vi "Paint Bounding Box (3).vi"(9 "Camera Image":T3, 10 "R/G/B":cluster{"Lower value":i32, "Upper value":i32}[](array[cluster])=[{"Lower value"=0, "Upper value"=40}, {"Lower value"=80, "Upper value"=255}, {"Lower value"=0, "Upper value"=255}]) -> (0 "Thresholded Image":T3(plugin-control), 1 "Bounding Box Final":T4, 2 "Particle Report 2":T1, 3 "Particle Report":T1, 4 "General Report":T2(array[cluster]))   [LabVIEW 2016]
uses:
  <vilib>/vision/Image Controls.llb/IMAQ Image.ctl
panel:
  out "Particle Report":T2(array[cluster]) {"Orientation" format="%.2f"; "Dimensions"."Height" format="%.2f"; "Dimensions"."Width" format="%.2f"; "Center of Mass"."Y" format="%.2f"; "Center of Mass"."X" format="%.2f"; "Bounding Rect"."Bottom" format="%.2f"; "Bounding Rect"."Right" format="%.2f"; "Bounding Rect"."Top" format="%.2f"; "Bounding Rect"."Left" format="%.2f"; "Number of Holes" format="%.2f"; "Area" format="%.2f"}
  in  "sampleimage":string
  out "Base Image":T3(plugin-control)
  # "difference = width*4"
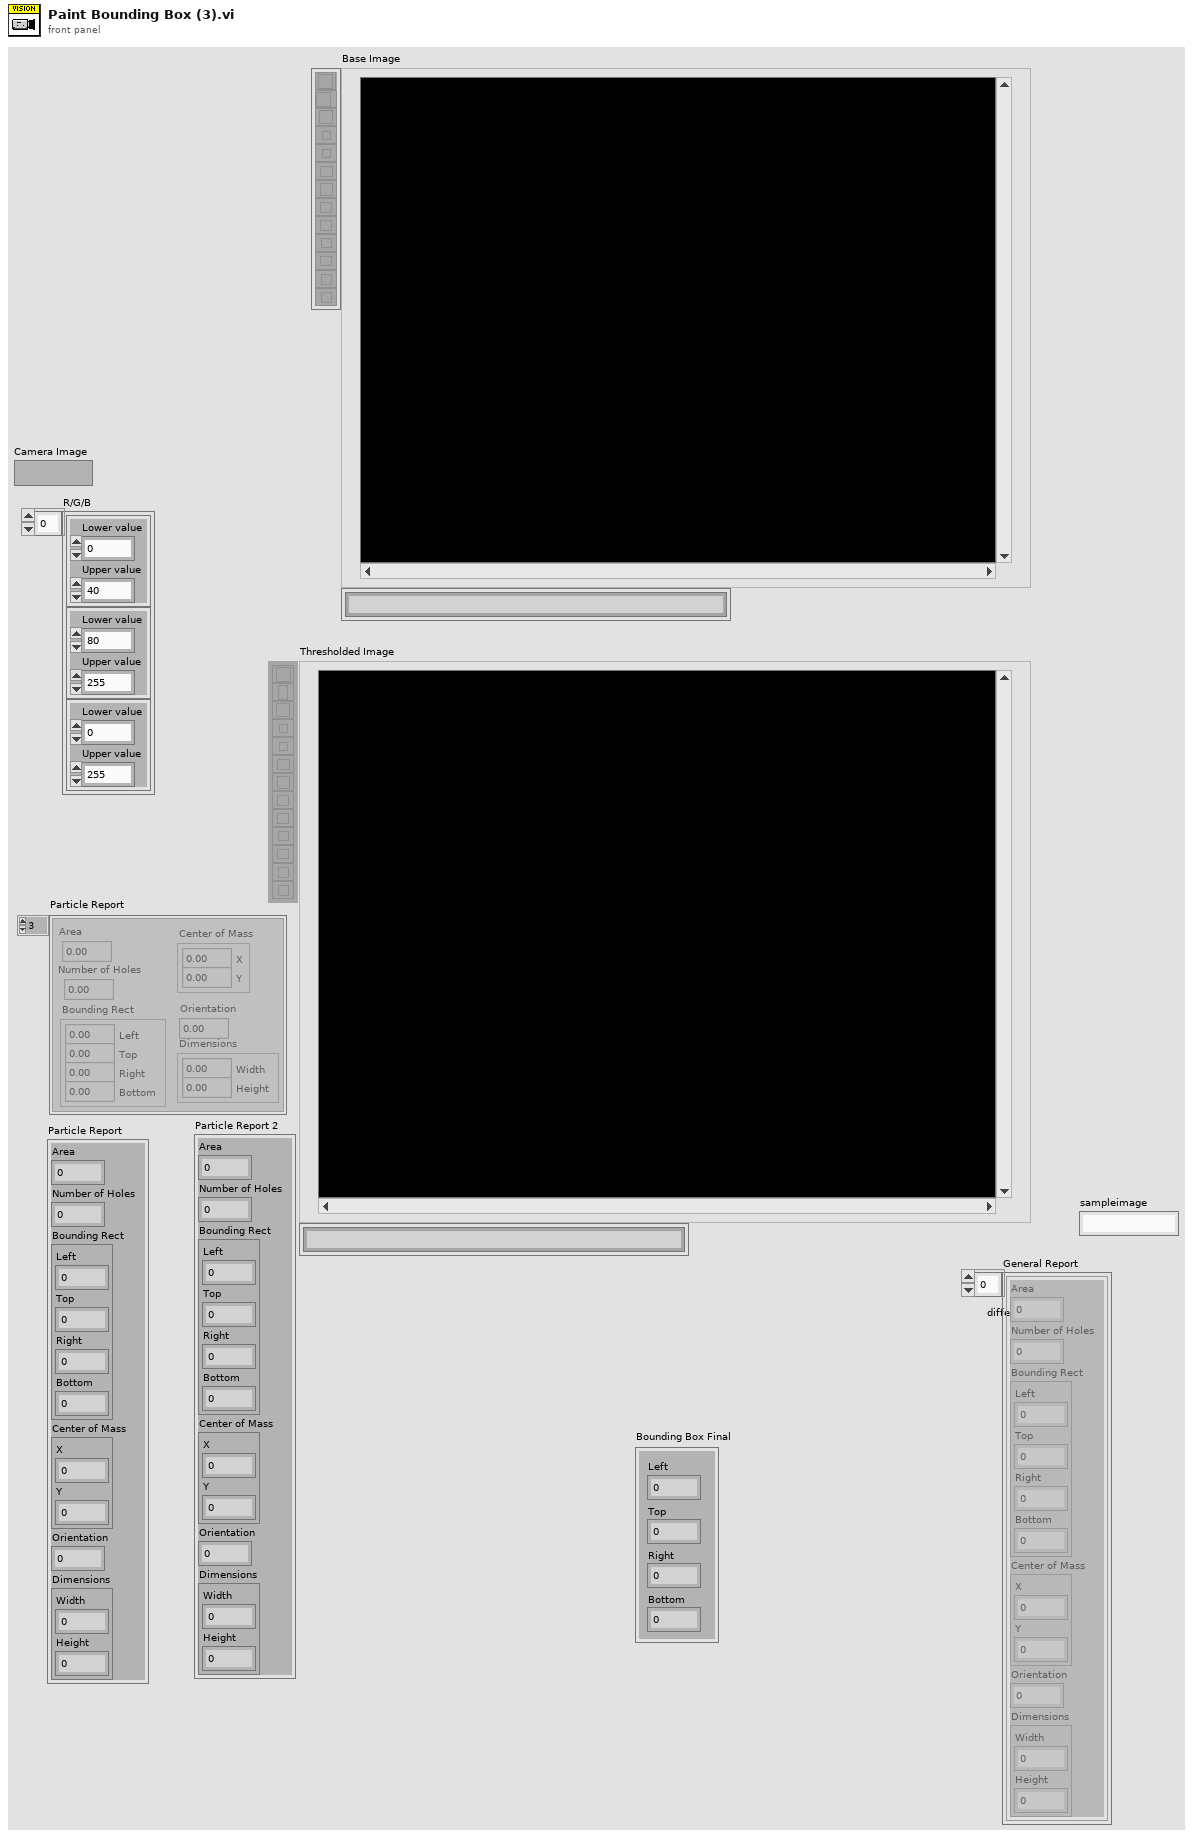
[diagram p1: front panel]
types:
  T1 = cluster{"Area":dbl, "Number of Holes":dbl, "Bounding Rect":cluster{"Left":dbl, "Top":dbl, "Right":dbl, "Bottom":dbl}, "Center of Mass":cluster{"X":dbl, "Y":dbl}, "Orientation":dbl, "Dimensions":cluster{"Width":dbl, "Height":dbl}}
  T2 = cluster{"Area":dbl, "Number of Holes":dbl, "Bounding Rect":cluster{"Left":dbl, "Top":dbl, "Right":dbl, "Bottom":dbl}, "Center of Mass":cluster{"X":dbl, "Y":dbl}, "Orientation":dbl, "Dimensions":cluster{"Width":dbl, "Height":dbl}}[]
  T3 = typedef "IMAQ Image.ctl" = refnum<image>
  T4 = cluster{"Left":dbl, "Top":dbl, "Right":dbl, "Bottom":dbl}
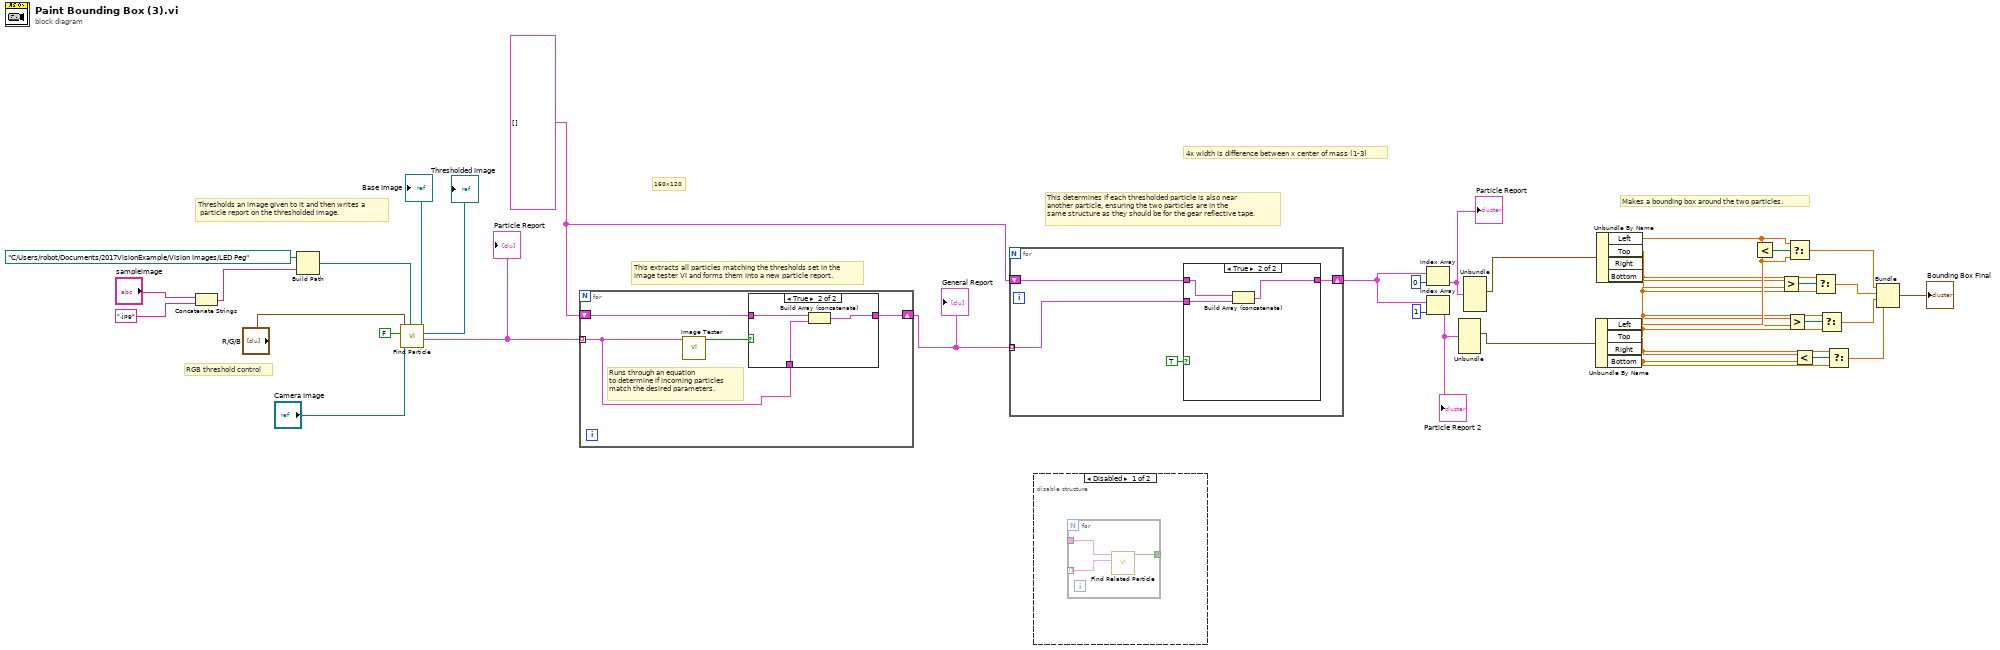
[diagram p0: block diagram]
diagram:
  w3 = T2 []
  # "This determines if each thresholded particle is also near \nanother particle, ensuring the two particles are in the \nsame structure as they should be for the gear reflective tape."
  # "Makes a bounding box around the two particles."
  # "4x width is difference between x center of mass (1-3)"
  # "RGB threshold control"
  # "This extracts all particles matching the thresholds set in the \nimage tester VI and forms them into a new particle report."
  # "Thresholds an image given to it and then writes a\n particle report on the thresholded image."
  # "160x120"
  n1 = Concatenate Strings("sampleimage", ".jpg" ("string")) -> (w28:string)
  n2 = Build Path(base path=path "C:/Users/robot/Documents/2017VisionExample/Vision Images/LED Peg", name or relative path=w28) -> (appended path=w29:path)
  n3 = call "Find Particle.vi"("File Path"=w29, "Camera Image"="Camera Image", "From File"=FALSE, "R/G/B"="R/G/B") -> ("Particle Report"=w35:T2, "Thresholded Image"=→"Thresholded Image":T3, "Base Image"=→"Base Image":T3)  [unwired: 3 in, 2 out]
  "Particle Report" <- w35
  n4 = for {
    tunnel: w35 -> [w38] mode=indexing
    shift-right: [w41] -> w4
    shift-left: w3 -> [w40]
    # "Runs through an equation\nto determine if incoming particles \nmatch the desired parameters."
    n5 = call "Image Tester.vi"("Particle Report"=w38) -> ("Positive"=w39:bool)  [unwired: 10 in]
    n6 = case shown="True" w39 {
      tunnel: w38 -> [_ w43]
      tunnel: [w42 w45] -> w41
      tunnel: w40 -> [w42 w44]
      frame False {
      }
      frame True {
        n7 = Build Array (concatenate)(w44, w43) -> (w45:T2)
      }
    }
  }
  "General Report" <- w4
  n8 = for {
    tunnel: w4 -> [w46] mode=indexing
    shift-right: [w49] -> w5
    shift-left: w3 -> [w48]
    n9 = case shown="True" TRUE {
      tunnel: [w50 w52] -> w49
      tunnel: w48 -> [w50 w53]
      tunnel: w46 -> [_ w51]
      frame False {
      }
      frame True {
        n10 = Build Array (concatenate)(w53, w51) -> (w52:T2)
      }
    }
  }
  n11 = disable-structure shown="Disabled" {
    frame Disabled {
      n12 = for {
        tunnel: _ -> [w56]
        tunnel: _ -> [w55] mode=indexing
        tunnel: [w54] -> _
        n13 = call "Find Related Particle.vi"("All Reports"=w55, "Base Report"=w56) -> ("Nearby"=w54:bool)  [unwired: 9 in]
      }
    }
    frame Enabled {
    }
  }
  n14 = Index Array(array=w5, index=0) -> (element=w25:T1)
  "Particle Report" <- w25
  n15 = Index Array(array=w5, index=1) -> (element=w24:T1)
  "Particle Report 2" <- w24
  n16 = Unbundle(w24) -> ("Bounding Rect"=w2:T4)  [unwired: 5 out]
  n17 = Unbundle(w25) -> ("Bounding Rect"=w1:T4)  [unwired: 5 out]
  n18 = Unbundle By Name(w2) -> ("Left"=w21:dbl, "Top"=w18:dbl, "Right"=w16:dbl, "Bottom"=w12:dbl)
  n19 = Unbundle By Name(w1) -> ("Left"=w22:dbl, "Top"=w19:dbl, "Right"=w15:dbl, "Bottom"=w13:dbl)
  n20 = Less?(x=w22, y=w21) -> (x < y?=w23:bool)
  n21 = Greater?(x=w19, y=w18) -> (0:w20:bool)
  n22 = Greater?(x=w15, y=w16) -> (0:w17:bool)
  n23 = Select(t=w22, s=w23, f=w21) -> (s? t:f=w11:dbl)
  n24 = Less?(x=w13, y=w12) -> (x < y?=w14:bool)
  n25 = Select(t=w19, s=w20, f=w18) -> (s? t:f=w10:dbl)
  n26 = Select(t=w15, s=w17, f=w16) -> (s? t:f=w9:dbl)
  n27 = Select(t=w13, s=w14, f=w12) -> (s? t:f=w8:dbl)
  n28 = Bundle("Left"=w11, "Top"=w10, "Right"=w9, "Bottom"=w8) -> (→"Bounding Box Final":T4)  [unwired: 1 in]
